vi "BayesianRidge.vi"(8 "error in":errorcluster) -> (0 "error out":errorcluster, 3 "out":refnum<class "BayesianRidge.lvclass">)   [LabVIEW 2020]
doc: "Bayesian ridge regression.\n\n Fit a Bayesian ridge model. See the Notes section for details on this\n implementation and the optimization of the regularization parameters\n lambda (precision of the weights) and alpha (precision of the noise).\n\n Read more in the :ref:`User Guide <bayesian_regression>`.\n\n Parameters\n ----------\n n_iter : int, default=300\n Maximum number of iterations. Should be greater than or equal to 1.\n\n tol : float, default=1e-3\n Stop the algorithm if w has converged.\n\n alpha_1 : float, default=1e-6\n Hyper-parameter : shape parameter for the Gamma distribution prior\n over the alpha parameter.\n\n alpha_2 : float, default=1e-6\n Hyper-parameter : inverse scale parameter (rate parameter) for the\n Gamma distribution prior over the alpha parameter.\n\n lambda_1 : float, default=1e-6\n Hyper-parameter : shape parameter for the Gamma distribution prior\n over the lambda parameter.\n\n lambda_2 : float, default=1e-6\n Hyper-parameter : inverse scale parameter (rate parameter) for the\n Gamma distribution prior over the lambda parameter.\n\n alpha_init : float, default=None\n Initial value for alpha (precision of the noise).\n If not set, alpha_init is 1/Var(y).\n\n .. versionadded:: 0.22\n\n lambda_init : float, default=None\n Initial value for lambda (precision of the weights).\n If not set, lambda_init is 1.\n\n .. versionadded:: 0.22\n\n compute_score : bool, default=False\n If True, compute the log marginal likelihood at each iteration of the\n optimization.\n\n fit_intercept : bool, default=True\n Whether to calculate the intercept for this model.\n The intercept is not treated as a probabilistic parameter\n and thus has no associated variance. If set\n to False, no intercept will be used in calculations\n (i.e. data is expected to be centered).\n\n normalize : bool, default=False\n This parameter is ignored when ``fit_intercept`` is set to False.\n If True, the regressors X will be normalized before regression by\n subtracting the mean and dividing by the l2-norm.\n If you wish to standardize, please use\n :class:`~sklearn.preprocessing.StandardScaler` before calling ``fit``\n on an estimator with ``normalize=False``.\n\n copy_X : bool, default=True\n If True, X will be copied; else, it may be overwritten.\n\n verbose : bool, default=False\n Verbose mode when fitting the model.\n\n\n Attributes\n ----------\n coef_ : array-like of shape (n_features,)\n Coefficients of the regression model (mean of distribution)\n\n intercept_ : float\n Independent term in decision function. Set to 0.0 if\n ``fit_intercept = False``.\n\n alpha_ : float\n Estimated precision of the noise.\n\n lambda_ : float\n Estimated precision of the weights.\n\n sigma_ : array-like of shape (n_features, n_features)\n Estimated variance-covariance matrix of the weights\n\n scores_ : array-like of shape (n_iter_+1,)\n If computed_score is True, value of the log marginal likelihood (to be\n maximized) at each iteration of the optimization. The array starts\n with the value of the log marginal likelihood obtained for the initial\n values of alpha and lambda and ends with the value obtained for the\n estimated alpha and lambda.\n\n n_iter_ : int\n The actual number of iterations to reach the stopping criterion.\n\n X_offset_ : float\n If `normalize=True`, offset subtracted for centering data to a\n zero mean.\n\n X_scale_ : float\n If `normalize=True`, parameter used to scale data to a unit\n standard deviation.\n\n \nAvailable methods:\nGet Attributes\nGet Params\nSet Params"
uses:
  BayesianRidge.lvclass
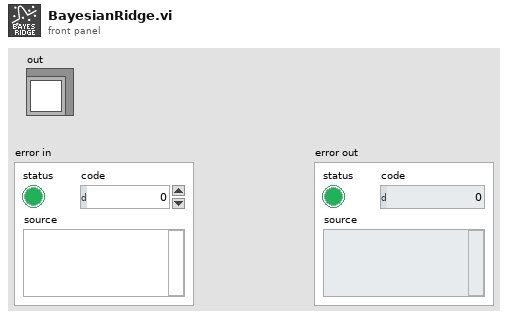
[diagram p1: front panel]
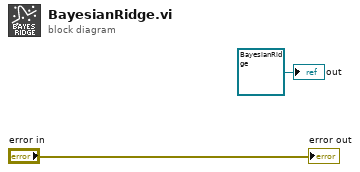
[diagram p0: block diagram]
diagram:
  "out" <- refnum<class "BayesianRidge.lvclass"> refnum ("model")
  "error out" <- "error in"
